vi "Create.vi"(8 "error in (no error)":errorcluster, 10 "thread configuration":T1, 11 "Thread Configuration in":refnum<class "Thread Configuration.lvclass">) -> (0 "error out":errorcluster, 3 "Thread Configuration out":refnum<class "Thread Configuration.lvclass">)   [LabVIEW 2017, in "DSF Core.lvlib" / "Thread Configuration.lvclass"]
uses:
  Thread Configuration.lvclass
  Group/Group Configuration.lvclass
  Runtime/Runtime Configuration.lvclass
  C:/Git/DSF/Core/Classes/Configuration/Runtime/Runtime Configuration.lvclass
  C:/Git/DSF/Core/Classes/Configuration/Configuration.lvclass
  Typedefs/DSF Settings Info.ctl
  DSF Core.lvlib
  Typedefs/DSF Engine Channel Configuration.ctl
  Typedefs/DSF Engine Transfer Configuration.ctl
  Typedefs/DSF Engine Transfer Group Configuration.ctl
  Typedefs/DSF Engine Plugin Thread Configuration.ctl
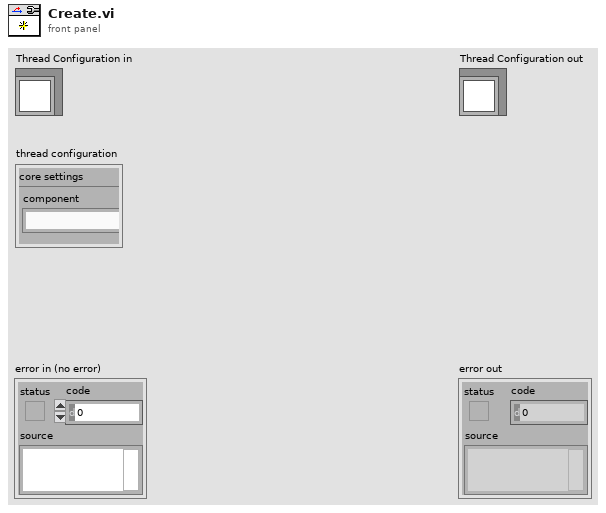
[diagram p1: front panel]
types:
  T1 = typedef "DSF Core.lvlib/DSF Engine Plugin Thread Configuration.ctl" = cluster{"core settings":T2, "component settings":T2[], "transfer groups":T3[]}
  T2 = typedef "DSF Core.lvlib/DSF Settings Info.ctl" = cluster{"component":string, "values":cluster{"key":string, "value":string}[]}
  T3 = typedef "DSF Core.lvlib/DSF Engine Transfer Group Configuration.ctl" = cluster{"core settings":T2, "component settings":T2[], "transfers":T4[]}
  T4 = typedef "DSF Core.lvlib/DSF Engine Transfer Configuration.ctl" = cluster{"core settings":T2, "component settings":T2[], "channels":T5[]}
  T5 = typedef "DSF Core.lvlib/DSF Engine Channel Configuration.ctl" = cluster{"core settings":T2, "component settings":T2[]}
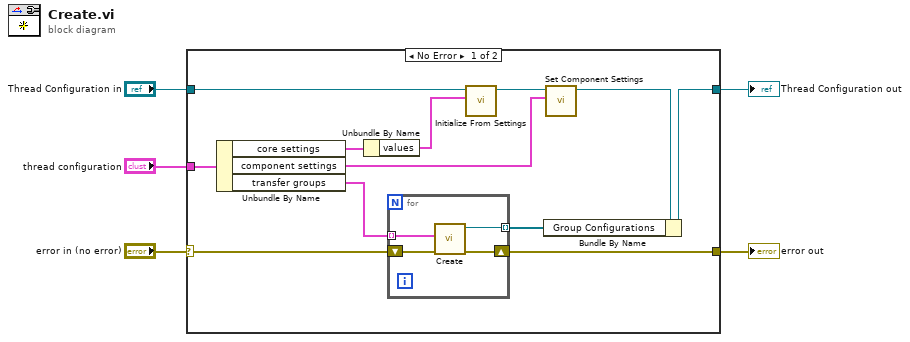
[diagram p0: block diagram]
diagram:
  n1 = case shown="No Error" "error in (no error)" {
    selector: "error in (no error)" -> [w16 w23]
    tunnel: [w13 w23] -> w4
    tunnel: [w17 w22] -> w2
    tunnel: "Thread Configuration in" -> [w9 w22]
    tunnel: "thread configuration" -> [w10 _]
    frame No Error {
      n2 = Unbundle By Name(w10) -> ("core settings"=w7:T2, "component settings"=w11:T2[], "transfer groups"=w15:T3[])
      n3 = Unbundle By Name(w7) -> ("values"=w6:cluster{"key":string, "value":string}[])
      n4 = for {
        shift-right: [w19] -> w13
        shift-left: w16 -> [w21]
        tunnel: w15 -> [w20] mode=indexing
        tunnel: [w18] -> w14 mode=indexing
        n5 = call "Create.vi"("error in (no error)"=w21, "group configuration"=w20) -> ("error out"=w19:errorcluster, "Group Configuration out"=w18:refnum<class "Group Configuration.lvclass">)  [unwired: 8 in]
      }
      n6 = call-dynamic "Initialize From Settings.vi"("settings"=w6, "Core Threads Configuration in"=w9) -> ("Core Threads Configuration out"=w8:refnum<class "Thread Configuration.lvclass">)  [unwired: 8 in, 1 out]
      n7 = call "Set Component Settings.vi"("component settings"=w11, "Runtime Configuration in"=w8) -> ("Runtime Configuration out"=w12:refnum<class "Thread Configuration.lvclass">)  [unwired: 8 in, 1 out]
      n8 = Bundle By Name(cluster=w12, "Group Configurations"=w14) -> (w17:refnum<class "Thread Configuration.lvclass">)
    }
    frame Error {
    }
  }
  "error out" <- w4
  "Thread Configuration out" <- w2
